vi "GetStraight EdgeResultNames.vi"(7 "ProjectName":string="Prj", 10 "Analysis_Find Straight Edge_Parameter":T1={"ROI Descriptor"={"Global Rectangle"=[], "Contours"=[]}, "Number of Matches Requested"=1, "Edge Info Size"=0, "Options"={"Search Direction"=0, "Edge Options"={"Edge Polarity"=0, "Kernel Size"=4, "Width"=3, "Minimum Edge Strength"=1024.0, "Interpolation Type"=enum."Zero Order", "Data Processing Method"=enum."Median"}, "Show Search Area"=FALSE, "Show Search Lines"=FALSE, "Show Edges Found"=FALSE, "Show Result"=TRUE, "Search Area Color"=5, "Search Lines Color"=3, "Edge Locations Color"=50, "Result Color"=1, "Overlay Group Name"=""}, "Line Fit Options"={"Number of Lines"=0, "Type"=enum."Best Edge Rake", "Min. Score"=0.0, "Max. Score"=25.0, "Orientation"=5.0, "Angle Range"=45.0, "Angle Tolerance"=1.0, "Step Size"=7, "Min. SNR (db)"=0.0, "Min. Points (%)"=25.0, "Hough Iterations"=5}} {"Line Fit Options"."Min. Points (%)" min=0.0 max=100.0; "Line Fit Options"."Min. SNR (db)" min=0.0; "Line Fit Options"."Max. Score" min=0.0 max=1024.0; "Line Fit Options"."Min. Score" min=0.0 max=1024.0 step=1.0; "Options"."Edge Options"."Edge Polarity" items=["All Edges", "Rising Edges", "Falling Edges"]; "Options"."Edge Options"."Minimum Edge Strength" format="%.2f"; "Options"."Edge Options"."Width" step=2; "Options"."Edge Options"."Kernel Size" step=2; "Options"."Search Direction" items=["Left to Right", "Right to Left", "Top to Bottom", "Bottom to Top"]}, 11 "ROI_Name":string="ROI1") -> (3 "ResultNames":string[](array[string]))   [LabVIEW 2019]
uses:
  Controls/Find Straight Edge/Analysis_Find Straight Edge_Result.ctl
  Controls/Find Straight Edge/Analysis_Find Straight Edge_Parameter.ctl
  <vilib>/vision/Measure.llb/Edge Options.ctl
  <vilib>/vision/Measure.llb/Edge Polarity.ctl
  <vilib>/vision/Measure.llb/Straight Edge Options.ctl
  <vilib>/vision/Measure.llb/Straight Edge Process.ctl
panel:
  in  "Analysis_Find Straight Edge_Result":T6={"ROI"={"Global Rectangle"=[27, 55, 270, 147], "Contours"=[{"Contour Type"=0, "ROI Type"=3, "Points"=[27, 55, 270, 147]}]}, "Number of Matches Requested"=1, "Straight Edges"=[]} {"Straight Edges"."Point2 (Real-World)"."Y" format="%.2f"; "Straight Edges"."Point2 (Real-World)"."X" format="%.2f"; "Straight Edges"."Point1 (Real-World)"."Y" format="%.2f"; "Straight Edges"."Point1 (Real-World)"."X" format="%.2f"; "Straight Edges"."Point2 (Pixels)"."Y" format="%.2f"; "Straight Edges"."Point2 (Pixels)"."X" format="%.2f"; "Straight Edges"."Point1 (Pixels)"."Y" format="%.2f"; "Straight Edges"."Point1 (Pixels)"."X" format="%.2f"; "Number of Matches Requested" min=1 max=9999}
  out "error out":errorcluster
  in  "error in (no error)":errorcluster
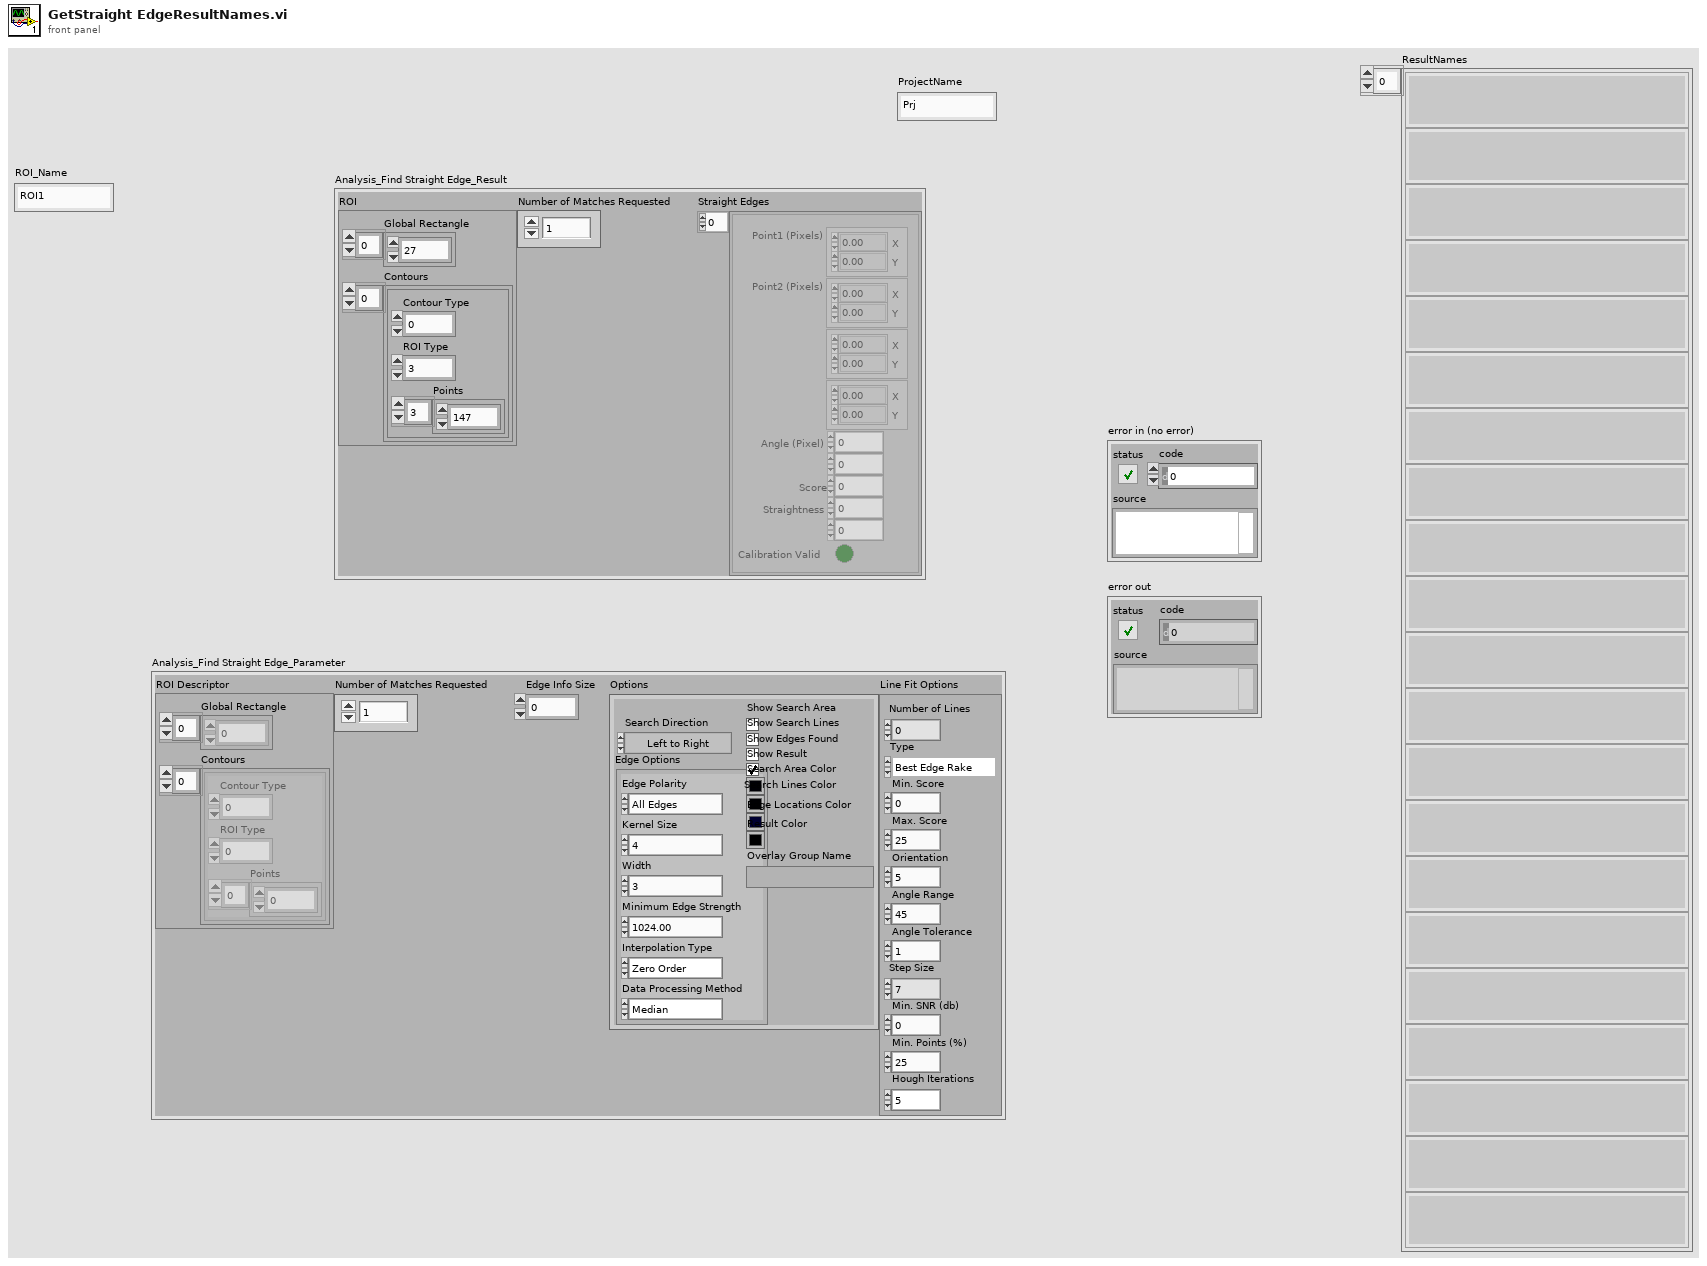
[diagram p1: front panel]
types:
  T1 = typedef "Analysis_Find Straight Edge_Parameter.ctl" = cluster{"ROI Descriptor":cluster{"Global Rectangle":i32[], "Contours":cluster{"Contour Type":u32, "ROI Type":u32, "Points":i32[]}[]}, "Number of Matches Requested":i32, "Edge Info Size":i32, "Options":cluster{"Search Direction":u32, "Edge Options":T2, "Show Search Area":bool, "Show Search Lines":bool, "Show Edges Found":bool, "Show Result":bool, "Search Area Color":u32, "Search Lines Color":u32, "Edge Locations Color":u32, "Result Color":u32, "Overlay Group Name":string}, "Line Fit Options":T4}
  T2 = typedef "Edge Options.ctl" = cluster{"Edge Polarity":T3, "Kernel Size":u32, "Width":u32, "Minimum Edge Strength":sgl, "Interpolation Type":enum32{"Zero Order", "Bilinear", "Quadratic", "Cubic", "Bilinear Fixed"}, "Data Processing Method":enum32{"Average", "Median"}}
  T3 = typedef "Edge Polarity.ctl" = u32
  T4 = typedef "Straight Edge Options.ctl" = cluster{"Number of Lines":i32, "Type":T5, "Min. Score":dbl, "Max. Score":dbl, "Orientation":dbl, "Angle Range":dbl, "Angle Tolerance":dbl, "Step Size":u32, "Min. SNR (db)":dbl, "Min. Points (%)":dbl, "Hough Iterations":i32}
  T5 = typedef "Straight Edge Process.ctl" = enum32{"First Edge Rake", "Best Edge Rake", "Hough Edge Rake", "First Edge Projection", "Best Edge Projection"}
  T6 = typedef "Analysis_Find Straight Edge_Result.ctl" = cluster{"ROI":cluster{"Global Rectangle":i32[], "Contours":cluster{"Contour Type":u32, "ROI Type":u32, "Points":i32[]}[]}, "Number of Matches Requested":i32, "Straight Edges":cluster{"Point1 (Pixels)":cluster{"X":sgl, "Y":sgl}, "Point2 (Pixels)":cluster{"X":sgl, "Y":sgl}, "Point1 (Real-World)":cluster{"X":sgl, "Y":sgl}, "Point2 (Real-World)":cluster{"X":sgl, "Y":sgl}, "Angle (Pixel)":dbl, "Angle (Real-World)":dbl, "Score":dbl, "Straightness":dbl, "Average SNR (db)":dbl, "Calibration Valid":bool}[]}
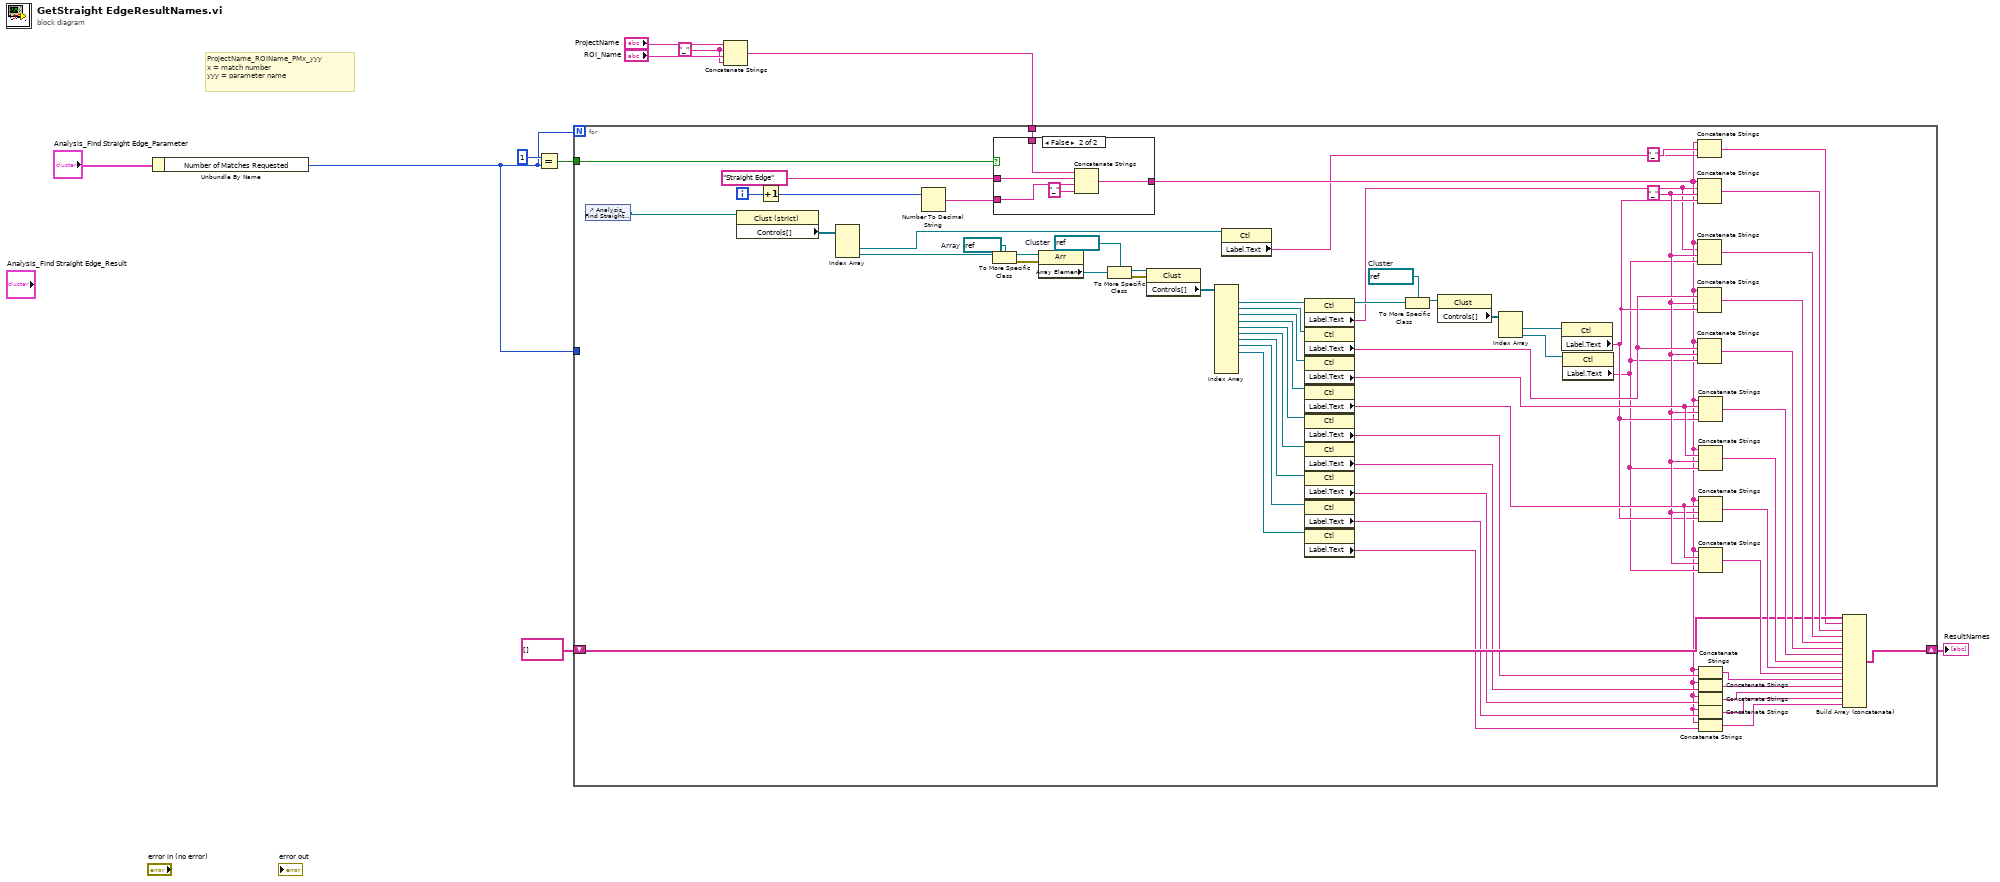
[diagram p0: block diagram]
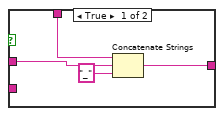
[diagram p2: hidden frame]
diagram:
  w8 = "_" ("string")
  # "ProjectName_ROIName_PMx_yyy\nx = match number\nyyy = parameter name"
  n1 = Unbundle By Name("Analysis_Find Straight Edge_Parameter") -> ("Number of Matches Requested"=w1:i32)
  n2 = Equal?(x=1, y=w1) -> (x = y?=w4:bool)
  n3 = Concatenate Strings("ProjectName", w8, "ROI_Name", w8) -> (w7:string)
  n4 = for {
    N: w1 -> [_]
    tunnel: w7 -> [w72]
    shift-right: [w29] -> w5
    shift-left: string[] [] -> [w28]
    tunnel: w4 -> [w73]
    tunnel: w1 -> [_]
    i -> [w69]
    w43 = "_" ("string")
    w51 = refnum<vi> refnum  # Cluster
    w62 = refnum<vi> refnum  # Cluster
    w66 = refnum<vi> refnum  # Array
    n5 = control-ref of="Analysis_Find Straight Edge_Result"() -> (w67:refnum<vi>)
    n6 = property class="Clust (strict)"(reference=w67) -> ("Controls[]"=w68:refnum<vi>[])  [unwired: 1 in, 2 out]
    n7 = Increment(x=w69) -> (x+1=w74:i32)
    n8 = Index Array(array=w68) -> (element #2=w11:refnum<vi>, element #3=w17:refnum<vi>)  [unwired: 3 in, 1 out]
    n9 = Number To Decimal String(number=w74) -> (decimal integer string=w71:string)  [unwired: 1 in]
    n10 = To More Specific Class(target class=w66, reference=w17) -> (specific class reference=w65:refnum<vi>, error out=w64:errorcluster)  [unwired: 1 in]
    n11 = case shown="False" w73 {
      tunnel: w72 -> [w78 w83]
      tunnel: w71 -> [_ w81]
      tunnel: [w77 w82] -> w15
      tunnel: "Straight Edge" ("string") -> [w76 w80]
      frame True {
        n12 = Concatenate Strings(w78, w76, "_" ("string")) -> (w77:string)
      }
      frame False {
        n13 = Concatenate Strings(w83, w80, w81, "_" ("string")) -> (w82:string)
      }
    }
    n14 = property class="Arr"(reference=w65, error in=w64) -> ("Array Element"=w63:refnum<vi>)  [unwired: 2 out]
    n15 = To More Specific Class(target class=w62, reference=w63) -> (specific class reference=w61:refnum<vi>, error out=w60:errorcluster)  [unwired: 1 in]
    n16 = property class="Clust"(reference=w61, error in=w60) -> ("Controls[]"=w59:refnum<vi>[])  [unwired: 2 out]
    n17 = Index Array(array=w59) -> (element #1=w58:refnum<vi>, element #2=w57:refnum<vi>, element #3=w56:refnum<vi>, element #4=w55:refnum<vi>, element #5=w54:refnum<vi>, element #6=w53:refnum<vi>, element #7=w32:refnum<vi>, element #8=w31:refnum<vi>, element #9=w30:refnum<vi>)  [unwired: 12 in, 3 out]
    n18 = property class="Ctl"(reference=w11) -> ("Label.Text"=w13:string)  [unwired: 1 in, 2 out]
    n19 = property class="Ctl"(reference=w58) -> (reference out=w52:refnum<vi>, "Label.Text"=w14:string)  [unwired: 1 in, 1 out]
    n20 = property class="Ctl"(reference=w57) -> ("Label.Text"=w46:string)  [unwired: 1 in, 2 out]
    n21 = property class="Ctl"(reference=w56) -> ("Label.Text"=w45:string)  [unwired: 1 in, 2 out]
    n22 = property class="Ctl"(reference=w55) -> ("Label.Text"=w44:string)  [unwired: 1 in, 2 out]
    n23 = property class="Ctl"(reference=w54) -> ("Label.Text"=w27:string)  [unwired: 1 in, 2 out]
    n24 = property class="Ctl"(reference=w53) -> ("Label.Text"=w26:string)  [unwired: 1 in, 2 out]
    n25 = property class="Ctl"(reference=w32) -> ("Label.Text"=w25:string)  [unwired: 1 in, 2 out]
    n26 = property class="Ctl"(reference=w31) -> ("Label.Text"=w24:string)  [unwired: 1 in, 2 out]
    n27 = property class="Ctl"(reference=w30) -> ("Label.Text"=w23:string)  [unwired: 1 in, 2 out]
    n28 = To More Specific Class(target class=w51, reference=w52) -> (specific class reference=w50:refnum<vi>)  [unwired: 1 in, 1 out]
    n29 = property class="Clust"(reference=w50) -> ("Controls[]"=w49:refnum<vi>[])  [unwired: 1 in, 2 out]
    n30 = Index Array(array=w49) -> (element #1=w48:refnum<vi>, element #2=w47:refnum<vi>)  [unwired: 2 in]
    n31 = property class="Ctl"(reference=w48) -> ("Label.Text"=w42:string)  [unwired: 1 in, 2 out]
    n32 = property class="Ctl"(reference=w47) -> ("Label.Text"=w41:string)  [unwired: 1 in, 2 out]
    n33 = Concatenate Strings(w15, "_" ("string"), w13) -> (w12:string)
    n34 = Concatenate Strings(w15, w14, w43, w42) -> (w40:string)
    n35 = Concatenate Strings(w15, w14, w43, w41) -> (w39:string)
    n36 = Concatenate Strings(w15, w46, w43, w42) -> (w38:string)
    n37 = Concatenate Strings(w15, w46, w43, w41) -> (w37:string)
    n38 = Concatenate Strings(w15, w45, w43, w42) -> (w36:string)
    n39 = Concatenate Strings(w15, w45, w43, w41) -> (w35:string)
    n40 = Concatenate Strings(w15, w44, w43, w42) -> (w34:string)
    n41 = Concatenate Strings(w15, w44, w43, w41) -> (w33:string)
    n42 = Concatenate Strings(w15, w27) -> (w22:string)
    n43 = Concatenate Strings(w15, w26) -> (w21:string)
    n44 = Concatenate Strings(w15, w25) -> (w20:string)
    n45 = Concatenate Strings(w15, w24) -> (w19:string)
    n46 = Concatenate Strings(w15, w23) -> (w18:string)
    n47 = Build Array (concatenate)(w28, w12, w40, w39, w38, w37, w36, w35, w34, w33, w22, w21, w20, w19, w18) -> (w29:string[])
  }
  "ResultNames" <- w5
